vi "Draw.vi"() -> ()   [LabVIEW 2019]
uses:
  States.ctl
  InputCluster.ctl
panel:
  in  "stop":bool
  in  "Index":dbl
  in  "Delete Point Index":bool
  in  "Delete last Point":bool
  in  "Accept Point":bool
  in  "X":dbl(slide) scale=0.0..10.0
  in  "Y":dbl(slide) scale=0.0..10.0
  out "XY Graph":dbl[][](graph)
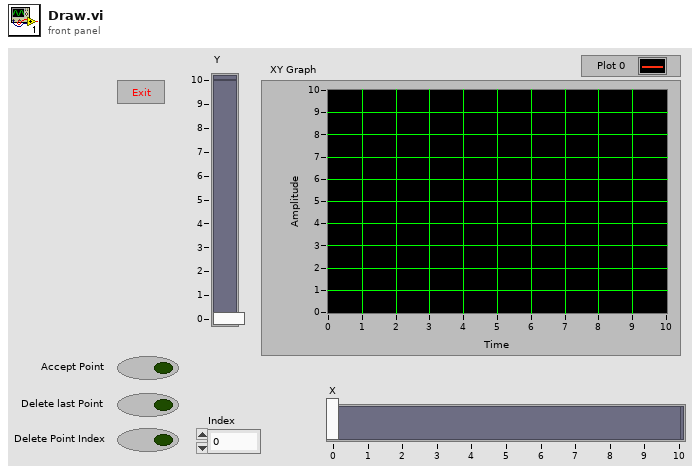
[diagram p1: front panel]
types:
  T1 = typedef "States.ctl" = enum16{"Init", "Idle", "Draw", "DeleteLastPoint", "DeletePointIndex", "Exit"}
  T2 = typedef "InputCluster.ctl" = cluster{"Value":dbl[][], "XValue":dbl, "Yvalue":dbl, "Index":dbl}
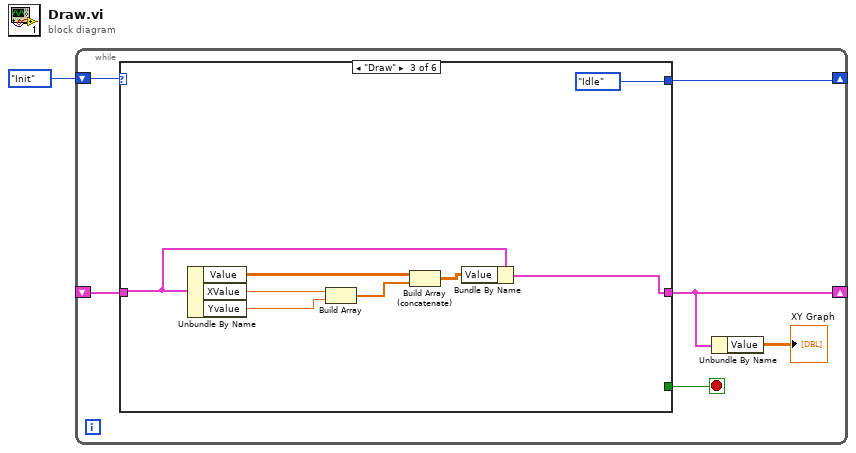
[diagram p0: block diagram]
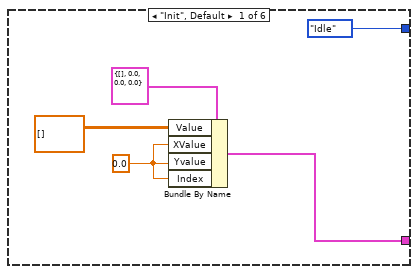
[diagram p2: hidden frame]
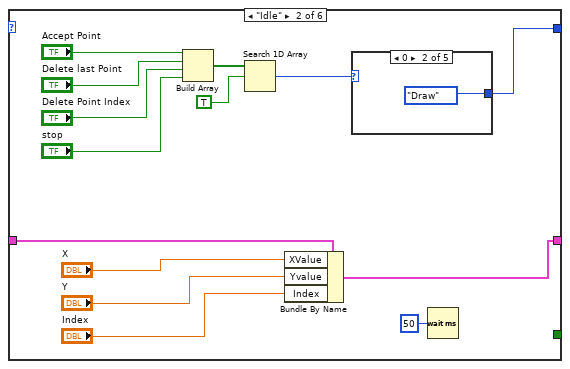
[diagram p3: hidden frame]
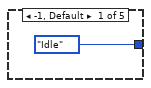
[diagram p4: hidden frame]
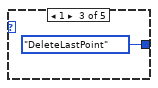
[diagram p5: hidden frame]
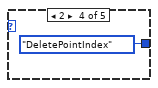
[diagram p6: hidden frame]
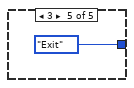
[diagram p7: hidden frame]
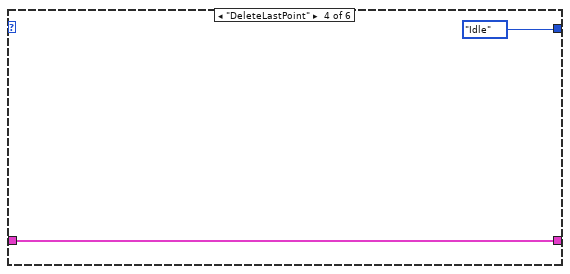
[diagram p8: hidden frame]
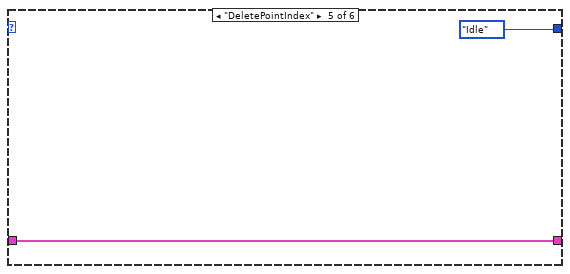
[diagram p9: hidden frame]
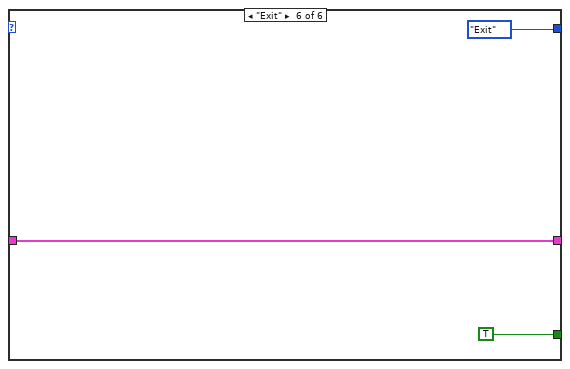
[diagram p10: hidden frame]
diagram:
  n1 = while {
    shift-right: [w4] -> _
    shift-left: _ -> [w6]
    shift-right: [w5] -> _
    shift-left: States."Init" -> [w7]
    stop <- w2 stop-if-true
    n2 = case shown="\"Draw\"" w7 {
      tunnel: [w11 w22 w34 w41 w43 w46] -> w4
      tunnel: w6 -> [_ w26 w35 w41 w43 w46]
      tunnel: [States."Idle" w13 States."Idle" States."Idle" States."Idle" States."Exit"] -> w5
      tunnel: [_ _ _ _ _ TRUE] -> w2
      frame "Init", Default {
        w9 = 0.0 ("Yvalue")
        n3 = Bundle By Name(cluster=T2 {"Value"=[], "XValue"=0.0, "Yvalue"=0.0, "Index"=0.0} ("Cluster"), "Value"=dbl[][] [], "XValue"=w9, "Yvalue"=w9, "Index"=w9) -> (w11:T2)
      }
      frame "Idle" {
        n4 = Build Array("Accept Point", "Delete last Point", "Delete Point Index", "stop") -> (w16:bool[])
        n5 = Search 1D Array(1D array=w16, element=TRUE) -> (index of element=w14:i32)  [unwired: 1 in]
        n6 = Bundle By Name(cluster=w26, "XValue"="X", "Yvalue"="Y", "Index"="Index") -> (w22:T2)
        n7 = case shown="0" w14 {
          tunnel: [States."Idle" States."Draw" States."DeleteLastPoint" States."DeletePointIndex" States."Exit"] -> w13
          frame -1, Default {
          }
          frame 0 {
          }
          frame 1 {
          }
          frame 2 {
          }
          frame 3 {
          }
        }
        n8 = Wait (ms)(milliseconds to wait=u32 50) -> ()  [unwired: 1 out]
      }
      frame "Draw" {
        n9 = Unbundle By Name(w35) -> ("Value"=w38:dbl[][], "XValue"=w33:dbl, "Yvalue"=w37:dbl)
        n10 = Build Array(w33, w37) -> (w32:dbl[])
        n11 = Build Array (concatenate)(w38, w32) -> (w36:dbl[][])
        n12 = Bundle By Name(cluster=w35, "Value"=w36) -> (w34:T2)
      }
      frame "DeleteLastPoint" {
      }
      frame "DeletePointIndex" {
      }
      frame "Exit" {
      }
    }
    n13 = Unbundle By Name(w4) -> ("Value"=→"XY Graph":dbl[][])
  }
